vi "Write SecurityKey.vi"(8 "error in (no error)":errorcluster, 10 "SecurityKey":bool[](array[boolean]), 11 "BB-Series in":refnum<class "BB-Series.lvclass">) -> (0 "error out":errorcluster, 3 "BB-Series out":refnum<class "BB-Series.lvclass">)   [LabVIEW 2021, in "BB-Series.lvclass"]
uses:
  BB-Series.lvclass
  BB-Series.lvclass/BB-Series.ctl
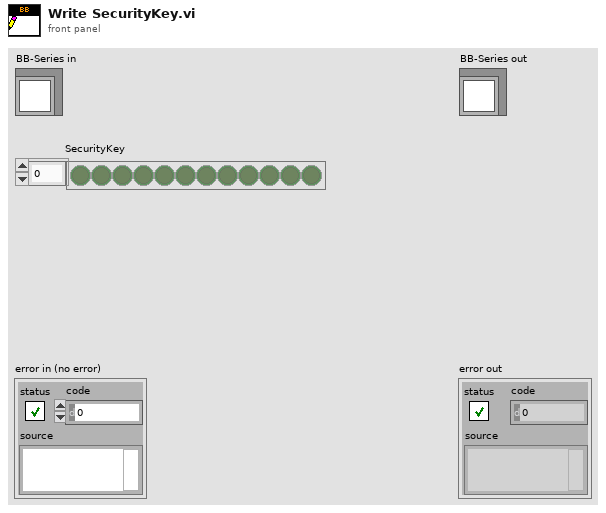
[diagram p1: front panel]
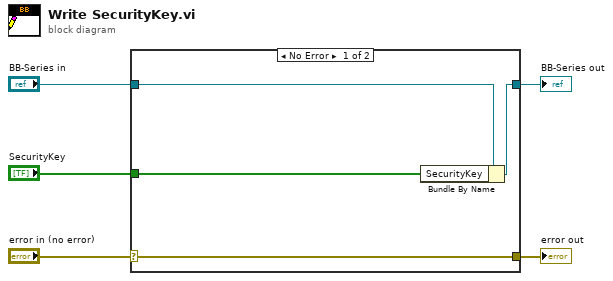
[diagram p0: block diagram]
diagram:
  n1 = case shown="No Error" "error in (no error)" {
    selector: "error in (no error)" -> [w9 w10]
    tunnel: [w9 w10] -> w4
    tunnel: [w7 w11] -> w2
    tunnel: "BB-Series in" -> [w8 w11]
    tunnel: "SecurityKey" -> [w6 _]
    frame No Error {
      n2 = Bundle By Name(cluster=w8, "SecurityKey"=w6) -> (w7:refnum<class "BB-Series.lvclass">)
    }
    frame Error {
    }
  }
  "error out" <- w4
  "BB-Series out" <- w2
